vi "SetPower.vi"(7 "Sync Group":u8=2 format="%08b", 8 "error in (no error)":errorcluster, 10 "MotorPower":dbl(slide) scale=-1.0..1.0, 11 "DriveMotorsLeft in":refnum<class "DriveMotorsLeft.lvclass">) -> (0 "error out":errorcluster, 3 "DriveMotorsLeft out":refnum<class "DriveMotorsLeft.lvclass">)   [LabVIEW 2013, in "DriveMotorsLeft.lvclass"]
uses:
  DriveMotorsLeft.lvclass
  DriveMotors/DriveMotors.lvclass
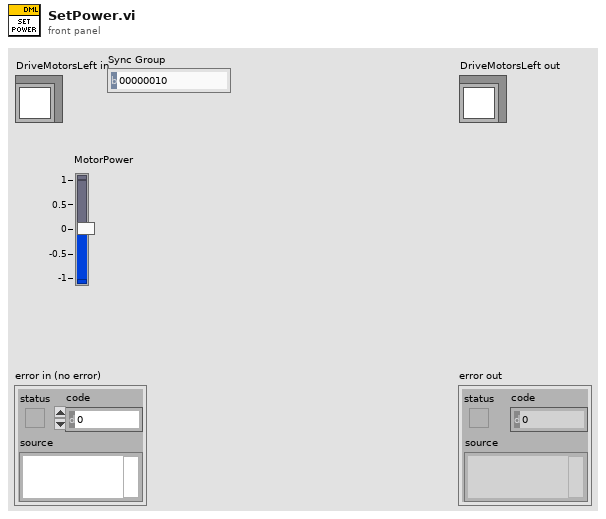
[diagram p1: front panel]
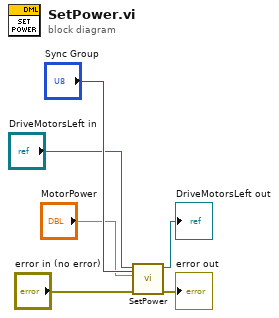
[diagram p0: block diagram]
diagram:
  n1 = call-parent "SetPower.vi"(7:"Sync Group", "error in (no error)"="error in (no error)", "MotorPower"="MotorPower", "DriveMotors in"="DriveMotorsLeft in") -> ("error out"=→"error out":errorcluster, "DriveMotors out"=→"DriveMotorsLeft out":refnum<class "DriveMotorsLeft.lvclass">)  [unwired: 6 in]
